vi "COM_TCP_01-telnet.vi"() -> ()   [LabVIEW 2025]
uses:
  <vilib>/platform/TimedLoop/XDataNode/XDataNode.xnode
  <vilib>/Platform/TimedLoop/XDataNode/nitl_modes.ctl
  <vilib>/Platform/TimedLoop/XDataNode/XDNodeRunTimeDep.lvlib
  <vilib>/Platform/TimedLoop/XDataNode/wakeup.ctl
  <vilib>/Platform/TimedLoop/XDataNode/timing_clust.ctl
panel:
  out "tension bateria":dbl
  out "bool sentido":dbl
  out "PWM motor":dbl
  out "corriente bateria":dbl
  out "distancia lidar lateral":dbl
  out "distancia lidar frontal":dbl
  out "angulo servo direccion":dbl
  in  "Enviar":bool
  out "Recibido":string="Inicio de comunicacion:"
  out "errCOM":errorcluster={"status"=TRUE, "code"=56, "source"="TCP Read in MB Ethernet Receive.vi:3100005->MB Ethernet Master Query.vi:2410004->MB Ethernet Master Query Write Multiple Coils (poly).vi->MBTCP_EJEMPLO_Master-simple.vi"}
  in  "Remote IP":string="192.168.137.47"
  in  "Remote Port":u16=23
  out "errorTX":errorcluster
  out "Enviados":u32
  in  "Escribe aquí":string
  in  "stop":bool
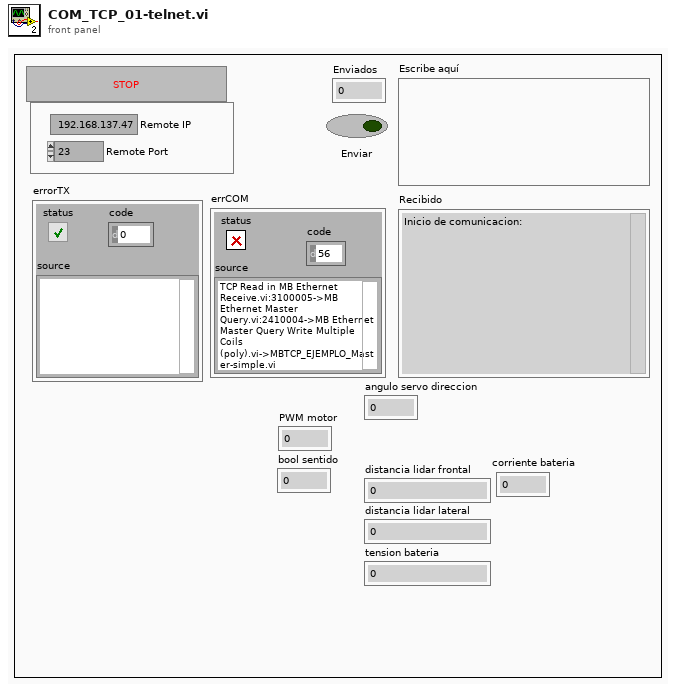
[diagram p1: front panel]
types:
  T1 = enum16{"Standard", "Buffered", "CRLF", "Immediate"}
  T2 = typedef "XDNodeRunTimeDep.lvlib/timing_clust.ctl" = cluster{"Expected End [f-1]":u64, "Actual End [f-1]":u64, "Finished Late? [f-1]":bool, "Expected End [i-1]":u64, "Actual End [i-1]":u64, "Finished Late? [i-1]":bool, "Expected Start [i]":u64, "Actual Start [i]":u64, "Expected Start [f]":u64, "Actual Start [f]":u64, "Source Name":string, "Structure Name":string, "Period":i64, "Deadline":i64, "Offset":i64, "Start":i64, "Priority":i32, "Timeout":i32, "Mode":T3, "Wakeup Reason":T4, "Error":errorcluster, "Source Type":string, "Secondary Source Type":string, "Global End Time":u64, "Global Start Time":u64, "Frame Duration":u64, "Iteration Duration":u64, "Assigned CPU":i32, "I/O Scan Engine Mode":u32}
  T3 = typedef "XDNodeRunTimeDep.lvlib/nitl_modes.ctl" = enum32{"No Change", "Process missed periods, maintain original phase", "Discard missed periods, maintain original phase", "Process missed periods, ignore original phase", "Discard missed periods, ignore original phase"}
  T4 = typedef "XDNodeRunTimeDep.lvlib/wakeup.ctl" = enum32{"Normal", "Aborted", "Asynchronous wakeup", "Timing source error", "Timed loop error", "Timeout"}
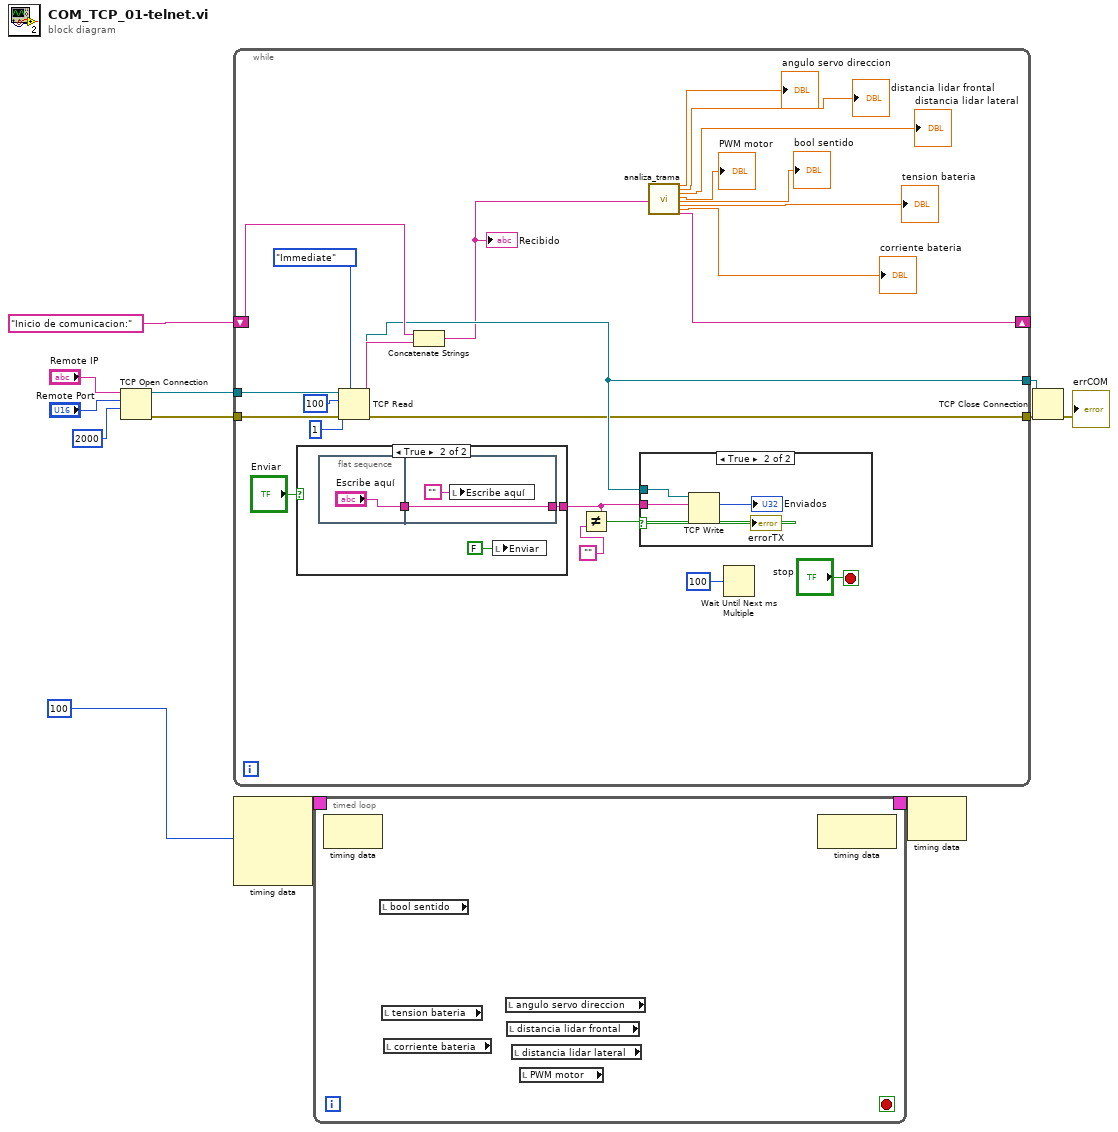
[diagram p0: block diagram]
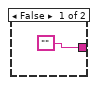
[diagram p2: hidden frame]
diagram:
  n1 = TCP Open Connection(address="Remote IP", remote port or service name="Remote Port", timeout ms (60000)=2000) -> (connection ID=w7:refnum<k5>, error out=w4:errorcluster)  [unwired: 1 in, 1 out]
  n2 = while {
    shift-right: [w21] -> _
    shift-left: "Inicio de comunicacion:" -> [w34]
    tunnel: w7 -> [w33]
    tunnel: [w29] -> w6
    tunnel: [w27] -> w5
    tunnel: w4 -> [w26]
    stop <- "stop" stop-if-true
    n3 = case shown="True" "Enviar" {
      tunnel: ["" w39] -> w25
      frame False {
      }
      frame True {
        n4 = flat-sequence {
          tunnel: ["Escribe aquí"] -> w40
          tunnel: [w43] -> w39
          tunnel: w40 -> [w43]
          frame #0 {
          }
          frame #1 {
            n5 = local write "Escribe aquí"("") -> ()
          }
        }
        n6 = local write "Enviar"(FALSE ("Enviar")) -> ()
      }
    }
    n7 = TCP Read(connection ID=w33, bytes to read=100, error in (no error)=w26, 7:T1."Immediate" ("mode (standard)"), 9:1 ("timeout ms (25000)")) -> (connection ID out=w29:refnum<k5>, data out=w30:string, error out=w27:errorcluster)
    n8 = Concatenate Strings(w34, w30) -> (w20:string)
    "Recibido" <- w20
    n9 = Not Equal?(x=w25, y="") -> (x != y?=w24:bool)
    n10 = case shown="True" w24 {
      tunnel: w25 -> [_ w47]
      tunnel: w29 -> [_ w46]
      frame False {
      }
      frame True {
        n11 = TCP Write(connection ID=w46, data in=w47) -> (bytes written=→"Enviados":i32, error out=→"errorTX":errorcluster)  [unwired: 2 in, 1 out]
      }
    }
    n12 = call "analiza_trama.vi"("Entrada"=w20) -> ("angulo servo direccion"=→"angulo servo direccion":dbl, "distancia lidar frontal"=→"distancia lidar frontal":dbl, "distancia lidar lateral"=→"distancia lidar lateral":dbl, "PWM motor"=→"PWM motor":dbl, "bool sentido"=→"bool sentido":dbl, "tension bateria"=→"tension bateria":dbl, "corriente bateria"=→"corriente bateria":dbl, "resto"=w21:string)  [unwired: 19 in]
    n13 = Wait Until Next ms Multiple(millisecond multiple=u32 100) -> ()  [unwired: 1 out]
  }
  n14 = node-c288(i64 100 ("Period")) -> (w3:T2)  [unwired: 3 in]
  n15 = timed-loop {
    timing: w3 -> [_]
    timing-out: [_] -> w2
    stop <- _ stop-if-true
    n16 = node-c288() -> ()  [unwired: 1 in, 1 out]
    n17 = local read "bool sentido"() -> ()  [unwired: 1 out]
    n18 = local read "tension bateria"() -> ()  [unwired: 1 out]
    n19 = local read "corriente bateria"() -> ()  [unwired: 1 out]
    n20 = local read "angulo servo direccion"() -> ()  [unwired: 1 out]
    n21 = local read "distancia lidar frontal"() -> ()  [unwired: 1 out]
    n22 = local read "distancia lidar lateral"() -> ()  [unwired: 1 out]
    n23 = local read "PWM motor"() -> ()  [unwired: 1 out]
    n24 = node-c288() -> ()  [unwired: 1 in, 1 out]
  }
  n25 = node-c288(w2) -> ()  [unwired: 1 out]
  n26 = TCP Close Connection(connection ID=w6, error in (no error)=w5) -> (error out=→"errCOM":errorcluster)  [unwired: 2 out]
